vi "Convert XY To Polar Velocities.vi"(11 "XY Velocities":T1) -> (3 "Polar Out":T2 {"Angle" scale format="%.3f"; "Velocity" scale=-1.0..1.0 scale format="%.1f"})   [LabVIEW 2023, in "Thor-SwerveDrive_ACT.lvlib"]
uses:
  Thor-SwerveDrive_ACT.lvlib
  Shared Code/TypeDefs/Cluster_Module Velocity-Direction-Rotations.ctl
  Shared Code/TypeDefs/Level_Velocity plus-minus 1.ctl
  Shared Code/TypeDefs/Dial_Compase heading unit circle CCW positive.ctl
  Shared Code/TypeDefs/Cluster_X-Y.ctl
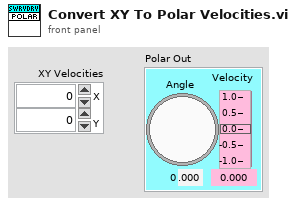
[diagram p1: front panel]
types:
  T1 = typedef "Cluster_X-Y.ctl" = cluster{"X":dbl, "Y":dbl}
  T2 = typedef "Cluster_Module Velocity-Direction-Rotations.ctl" = cluster{"Velocity":T3, "Angle":T4, "Rotations Count":dbl}
  T3 = typedef "Level_Velocity plus-minus 1.ctl" = dbl
  T4 = typedef "Dial_Compase heading unit circle CCW positive.ctl" = dbl
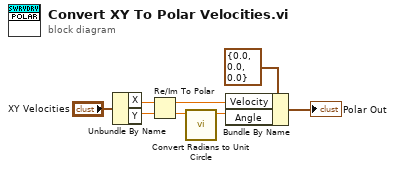
[diagram p0: block diagram]
diagram:
  n1 = Unbundle By Name("XY Velocities") -> ("X"=w8:dbl, "Y"=w4:dbl)
  n2 = Re/Im To Polar(2:w4, 3:w8) -> (0:w3:dbl, 1:w7:dbl)
  n3 = call "Convert Radians to Unit Circle.vi"("Radians"=w3) -> ("Unit Circle"=w2:dbl)  [unwired: 10 in]
  n4 = Bundle By Name(cluster=T2 {"Velocity"=0.0, "Angle"=0.0, "Rotations Count"=0.0} ("Polar Out"), "Velocity"=w7, "Angle"=w2) -> (→"Polar Out":T2)
